vi "record.vi"(0 "Camera in":refnum<class "Camera.lvclass">, 5 "num_images":u32=1, 7 "record_mode":T1(ring), 9 "file_path":path, 11 "error in (no error)":errorcluster, 12 "wFlags":u16 format="%04x") -> (4 "Camera out":refnum<class "Camera.lvclass">, 15 "error out":errorcluster)   [LabVIEW 2019, in "Camera.lvclass"]
doc: "Creates, configures, and starts a new recorder instance. The entire camera configuration must be\nset before calling record.vi. The VI's for getting and setting delay/exposure time are the only exception.\nThese functions have no effect on the recorder object and can be called during the recording."
uses:
  Camera.lvclass
  Camera.lvclass/Camera.ctl
  pco.recorder/Recorder.lvlib
  pco.sdk/RecordingControl/RecordingControl.lvlib
  pco.sdk/ImageSensor/ImageSensor.lvlib
  pco.convert/Convert.lvlib
panel:
  out "filemode_no_overwrite":bool
  out "blocking_int":bool
  out "recType_int":u16
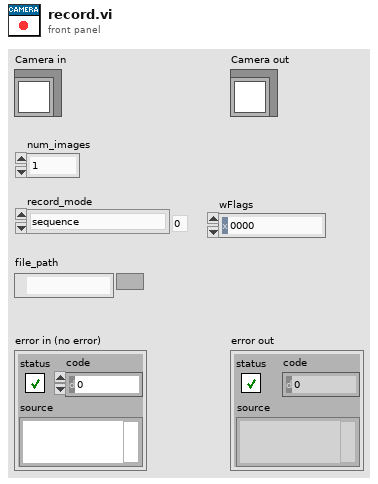
[diagram p1: front panel]
types:
  T1 = enum16{"sequence", "sequence non blocking", "ring buffer", "fifo", "tif", "multitif", "pcoraw", "b16", "dicom", "multidicom", "camram_ring", "camram_segment"}
  T2 = map{enum16{"Undefined", "Mono8", "Mono16", "BGRA8", "RGBA8", "BGRA16", "RGBA16", "CompressedMono8"}, bool}
  T3 = cluster{"wSensorTypeDESC":u16, "wSensorSubTypeDESC":u16, "wMaxHorzResStdDESC":u16, "wMaxVertResStdDESC":u16, "wMaxHorzResExtDESC":u16, "wMaxVertResExtDESC":u16, "wDynResDESC":u16, "wMaxBinHorzDESC":u16, "wBinHorzSteppingDESC":u16, "wMaxBinVertDESC":u16, "wBinVertSteppingDESC":u16, "wRoiHorStepsDESC":u16, "wRoiVertStepsDESC":u16, "wNumADCsDESC":u16, "wMinSizeHorzDESC":u16, "dwPixelRateDESC":u32[], "wConvFactDESC":u16[], "sCoolingSetpoints":i16[], "wSoftRoiHorStepsDESC":u16, "wSoftRoiVertStepsDESC":u16, "wIRDESC":u16, "wMinSizeVertDESC":u16, "dwMinDelayDESC":u32, "dwMaxDelayDESC":u32, "dwMinDelayStepDESC":u32, "dwMinExposureDESC":u32, "dwMaxExposureDESC":u32, "dwMinExposureStepDESC":u32, "dwMinDelayIRDESC":u32, "dwMaxDelayIRDESC":u32, "dwMinExposureIRDESC":u32, "dwMaxExposureIRDESC":u32, "wTimeTableDESC":u16, "wDoubleImageDESC":u16, "sMinCoolSetDESC":i16, "sMaxCoolSetDESC":i16, "sDefaultCoolSetDESC":i16, "wPowerDownModeDESC":u16, "wOffsetRegulationDESC":u16, "wColorPatternDESC":u16, "wPatternTypeDESC":u16, "wNumCoolingSetpoints":u16, "dwGeneralCapsDESC1":u32, "dwGeneralCapsDESC2":u32, "dwExtSyncFrequency":u32[], "dwGeneralCapsDESC3":u32, "dwGeneralCapsDESC4":u32}
  T4 = cluster{"iConversionFactor":i32, "iDataBits":i32, "iSensorInfoBits":i32, "iDarkOffset":i32, "strColorCoeff":dbl[], "iCamNum":i32, "hCamera":u64}
  T5 = map{enum16{"Undefined", "Mono8", "Mono16", "BGRA8", "RGBA8", "BGRA16", "RGBA16", "CompressedMono8"}, u64}
  T6 = enum16{"Undefined", "Mono8", "Mono16", "BGRA8", "RGBA8", "BGRA16", "RGBA16", "CompressedMono8"}
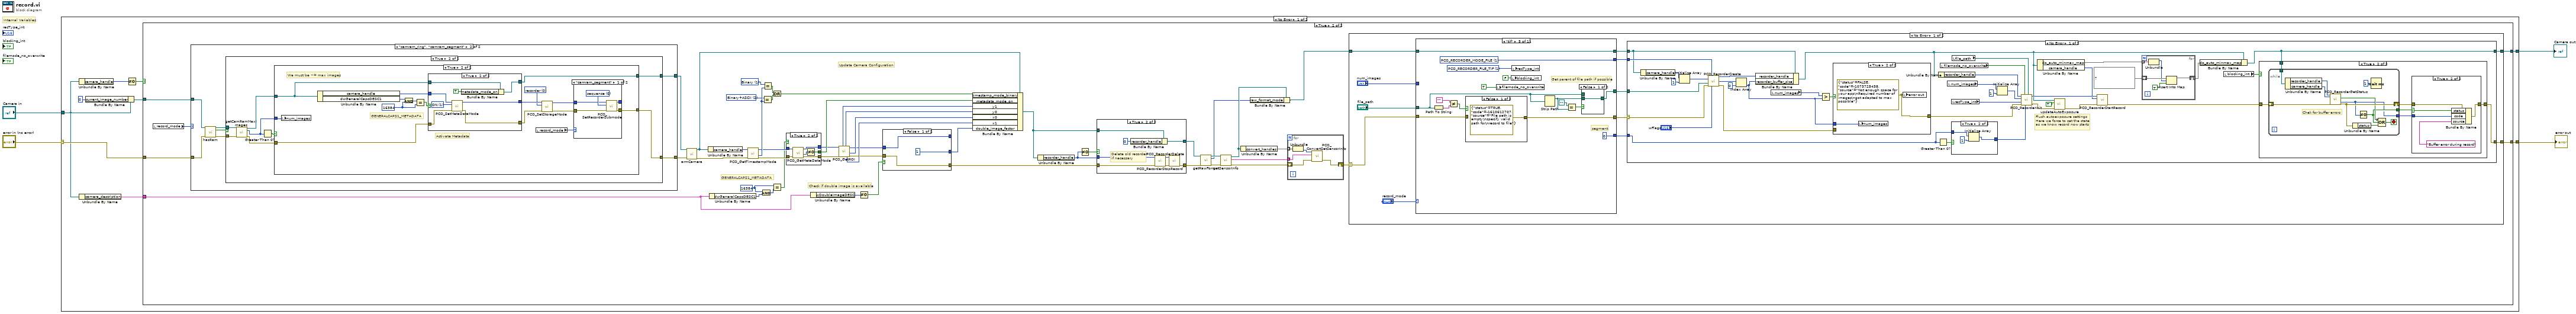
[diagram p0: block diagram]
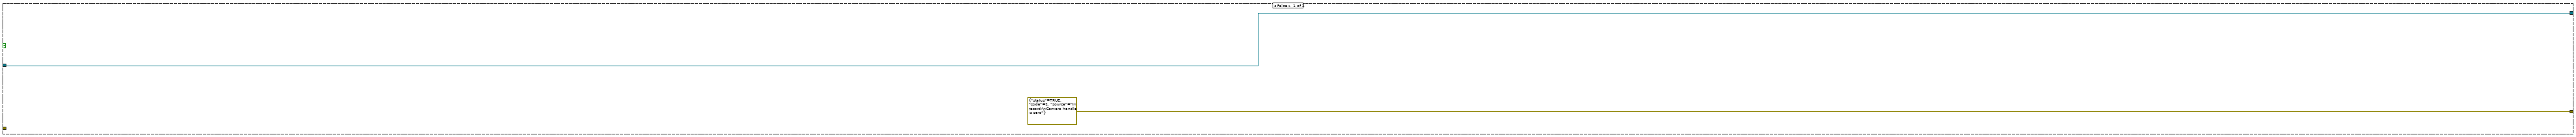
[diagram p2: hidden frame]
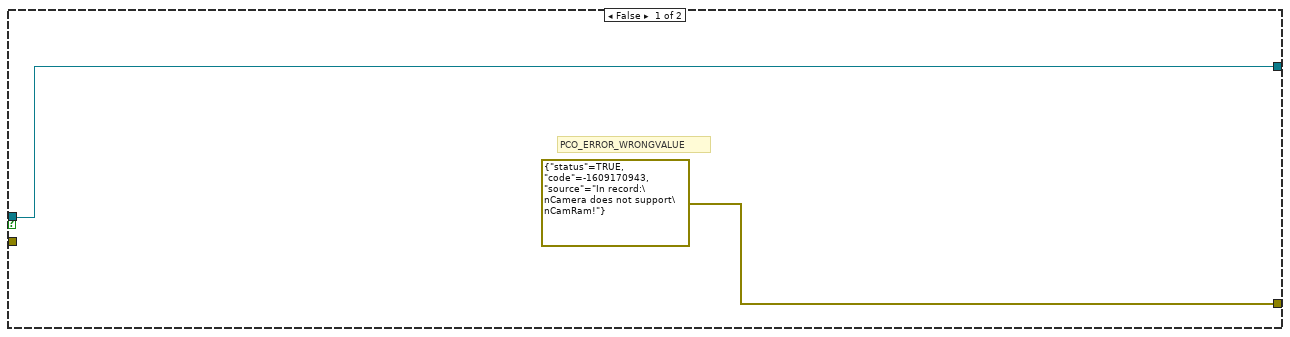
[diagram p4: hidden frame]
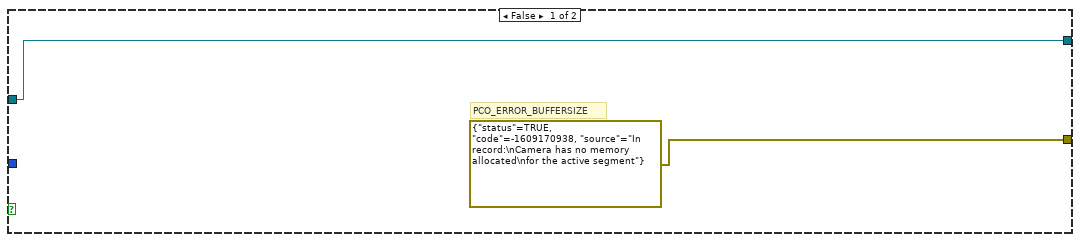
[diagram p5: hidden frame]
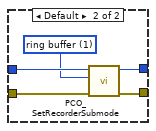
[diagram p6: hidden frame]
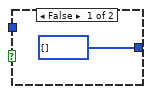
[diagram p8: hidden frame]
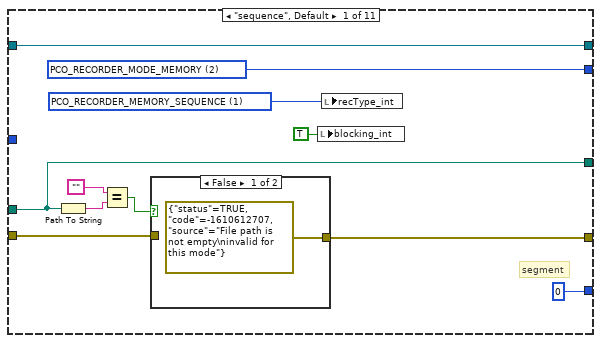
[diagram p13: hidden frame]
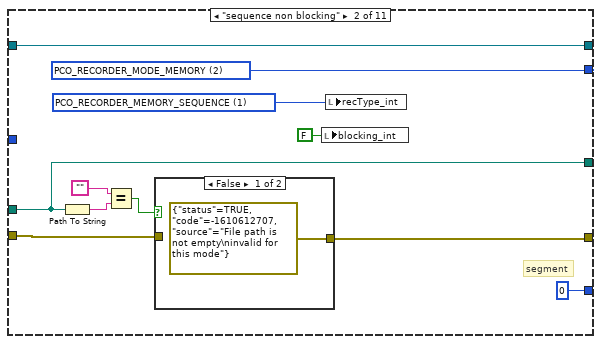
[diagram p15: hidden frame]
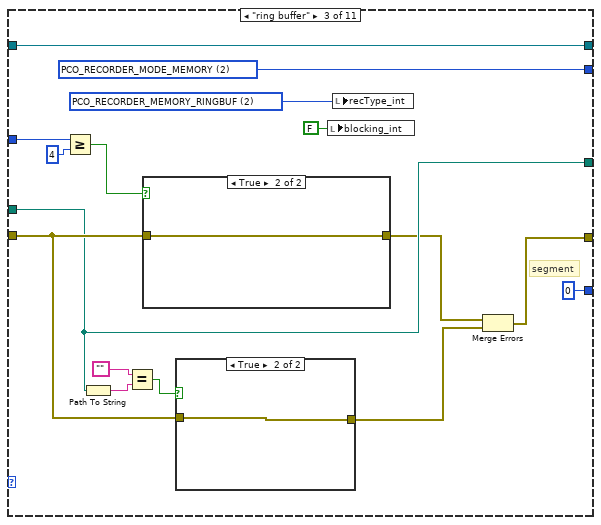
[diagram p17: hidden frame]
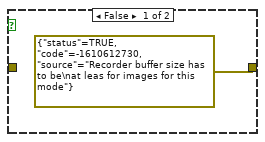
[diagram p18: hidden frame]
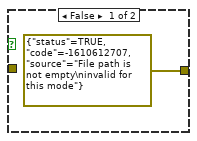
[diagram p19: hidden frame]
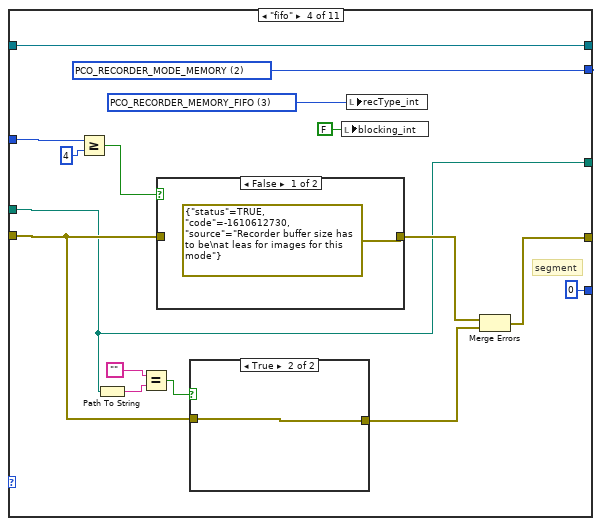
[diagram p20: hidden frame]
diagram:
  # "Internal Variables"
  n1 = case shown="No Error" "error in (no error)" {
    selector: "error in (no error)" -> [w9 w453]
    tunnel: [w12 w453] -> w3
    tunnel: [w11 w452] -> w1
    tunnel: "Camera in" -> [w7 w452]
    frame No Error {
      n2 = Unbundle By Name(w7) -> ("camera_handle"=w10:u64)
      n3 = Unbundle By Name(w7) -> ("camera_description"=w8:T3)
      n4 = Bundle By Name(cluster=w7, "current_image_number"=u32 0) -> (w6:refnum<class "Camera.lvclass">)
      n5 = Not Equal To 0?(x=w10) -> (x != 0?=w13:bool)
      n6 = case shown="True" w13 {
        tunnel: [errorcluster {"status"=TRUE, "code"=1, "source"="In record:\nCamera handle is zero"} ("error constant") w32] -> w12
        tunnel: w9 -> [_ w29]
        tunnel: w6 -> [w14 w27]
        tunnel: [w14 w31] -> w11
        tunnel: w8 -> [_ w45]
        frame False {
        }
        frame True {
          w54 = u32 16384 ("dwGeneralCapsDESC1")
          w62 = u16 2 items=["OFF", "Binary", "Binary+ASCII", "ASCII"] ("wTimeStampMode")
          w64 = u16 1 items=["OFF", "Binary", "Binary+ASCII", "ASCII"] ("wTimeStampMode")
          # "Update Camera Configuration"
          # "Check if double image is available"
          # "GENERALCAPS1_METADATA"
          n7 = local read "record_mode"() -> (w30:T1)
          n8 = case shown="\"camram_ring\", \"camram_segment\"" w30 {
            tunnel: w29 -> [w67 w72]
            tunnel: [w67 w68] -> w28
            tunnel: w27 -> [w66 w73]
            tunnel: [w66 w69] -> w18
            frame Default {
            }
            frame "camram_ring", "camram_segment" {
              n9 = call-dynamic "hasRam.vi"("Camera in"=w73, "error in (no error)"=w72) -> ("Camera out"=w70:refnum<class "Camera.lvclass">, "hasRam"=w74:bool, "error out"=w71:errorcluster)  [unwired: 11 in]
              n10 = case shown="True" w74 {
                tunnel: w71 -> [_ w83]
                tunnel: w70 -> [w76 w84]
                tunnel: [w76 w78] -> w69
                tunnel: [errorcluster {"status"=TRUE, "code"=-1609170943, "source"="In record:\nCamera does not support\nCamRam!"} ("error constant") w77] -> w68
                frame False {
                  # "PCO_ERROR_WRONGVALUE"
                }
                frame True {
                  n11 = call-dynamic "getCamRamMaxImages.vi"("Camera in"=w84, "error in (no error)"=w83) -> ("Camera out"=w80:refnum<class "Camera.lvclass">, "max_images"=w79:u32, "error out"=w81:errorcluster)  [unwired: 11 in]
                  n12 = Greater Than 0?(x=w79) -> (x > 0?=w82:bool)
                  n13 = case shown="True" w82 {
                    tunnel: w81 -> [_ w97]
                    tunnel: w80 -> [w86 w96]
                    tunnel: w79 -> [_ w87]
                    tunnel: [w86 w89] -> w78
                    tunnel: [errorcluster {"status"=TRUE, "code"=-1609170938, "source"="In record:\nCamera has no memory allocated\nfor the active segment"} ("error constant") w88] -> w77
                    frame False {
                      # "PCO_ERROR_BUFFERSIZE"
                    }
                    frame True {
                      w93 = u16 0 items=["recorder", "FIFO buffer"] ("wStorageMode")
                      w101 = u32 16384 ("y")
                      # "Activate Metadata"
                      # "GENERALCAPS1_METADATA"
                      # "We must be <= max images"
                      n14 = local write "num_images"(w87) -> ()
                      n15 = Unbundle By Name(w96) -> ("camera_handle"=w98:u64, "dwGeneralCapsDESC1"=w100:u32)
                      n16 = And(x=w100, y=w101) -> (x .and. y?=w102:u32)
                      n17 = Equal?(x=w102, y=w101) -> (x = y?=w99:bool)
                      n18 = case shown="True" w99 {
                        tunnel: w98 -> [w114 w123]
                        tunnel: w97 -> [w115 w122]
                        tunnel: w96 -> [w113 w120]
                        tunnel: [w113 w118] -> w89
                        tunnel: [w115 w117] -> w94
                        tunnel: [w114 w116] -> w95
                        frame False {
                        }
                        frame True {
                          w121 = u16 1 items=["OFF", "ON"] ("wMetaDataMode")
                          n19 = call "PCO_SetMetaDataMode.vi"("error in (no error)"=w122, "wMetaDataMode"=w121, "ph"=w123) -> ("error out"=w117:errorcluster, "ph out"=w116:u64)  [unwired: 4 in, 3 out]
                          n20 = Bundle By Name(cluster=w120, "metadata_mode_on"=TRUE) -> (w118:refnum<class "Camera.lvclass">)
                        }
                      }
                      n21 = local read "record_mode"() -> (w92:T1)
                      n22 = call "PCO_SetStorageMode.vi"("error in (no error)"=w94, "wStorageMode"=w93, "ph"=w95) -> ("error out"=w91:errorcluster, "ph out"=w90:u64)  [unwired: 6 in, 1 out]
                      n23 = case shown="\"camram_segment\"" w92 {
                        tunnel: w91 -> [w105 w111]
                        tunnel: w90 -> [w106 w112]
                        tunnel: [w104 w109] -> _
                        tunnel: [w103 w108] -> w88
                        frame "camram_segment" {
                          w107 = u16 0 items=["sequence", "ring buffer"] ("wRecSubmode")
                          n24 = call "PCO_SetRecorderSubmode.vi"("error in (no error)"=w105, "wRecSubmode"=w107, "ph"=w106) -> ("error out"=w103:errorcluster, "ph out"=w104:u64)  [unwired: 6 in, 1 out]
                        }
                        frame Default {
                          w110 = u16 1 items=["sequence", "ring buffer"] ("wRecSubmode")
                          n25 = call "PCO_SetRecorderSubmode.vi"("error in (no error)"=w111, "wRecSubmode"=w110, "ph"=w112) -> ("error out"=w108:errorcluster, "ph out"=w109:u64)  [unwired: 6 in, 1 out]
                        }
                      }
                    }
                  }
                }
              }
            }
          }
          n26 = call-dynamic "armCamera.vi"("Camera in"=w18, "error in (no error)"=w28) -> ("Camera out"=w16:refnum<class "Camera.lvclass">, "error out"=w65:errorcluster)  [unwired: 12 in]
          n27 = Unbundle By Name(w16) -> ("camera_handle"=w17:u64)
          n28 = Unbundle By Name(w45) -> ("dwGeneralCapsDESC1"=w56:u32)
          n29 = call "PCO_GetTimestampMode.vi"("error in (no error)"=w65, "ph"=w17) -> ("error out"=w57:errorcluster, "wTimeStampMode"=w63:u16, "ph out"=w58:u64)  [unwired: 6 in, 1 out]
          n30 = And(x=w54, y=w56) -> (x .and. y?=w55:u32)
          n31 = Equal?(x=w62, y=w63) -> (x = y?=w61:bool)
          n32 = Equal?(x=w64, y=w63) -> (x = y?=w60:bool)
          n33 = Or(x=w60, y=w61) -> (x .or. y?=w59:bool)
          n34 = Equal?(x=w54, y=w55) -> (x = y?=w53:bool)
          n35 = case shown="True" w53 {
            tunnel: w58 -> [w443 w451]
            tunnel: w57 -> [w444 w450]
            tunnel: [w443 w449] -> w51
            tunnel: [w444 w448] -> w50
            tunnel: [FALSE w446] -> w52
            frame False {
            }
            frame True {
              n36 = call "PCO_GetMetaDataMode.vi"("error in (no error)"=w450, "ph"=w451) -> ("error out"=w448:errorcluster, "wMetaDataMode"=w447:u16, "ph out"=w449:u64)  [unwired: 4 in, 3 out]
              n37 = Not Equal To 0?(x=w447) -> (x != 0?=w446:bool)
            }
          }
          n38 = Unbundle By Name(w45) -> ("wDoubleImageDESC"=w44:u16)
          n39 = call "PCO_GetROI.vi"("error in (no error)"=w50, "ph"=w51) -> ("error out"=w42:errorcluster, "wRoiX0"=w47:u16, "ph out"=w41:u64, "wRoiX1"=w46:u16, "wRoiY0"=w49:u16, "wRoiY1"=w48:u16)  [unwired: 3 in, 1 out]
          n40 = Not Equal To 0?(x=w44) -> (x != 0?=w43:bool)
          n41 = case shown="False" w43 {
            tunnel: w42 -> [w431 w440]
            tunnel: w41 -> [w432 w439]
            tunnel: [u16 1 ("double_image_factor") w436] -> w40
            tunnel: [w431 w435] -> w39
            tunnel: [w432 w434] -> _
            frame False {
            }
            frame True {
              n42 = call "PCO_GetDoubleImageMode.vi"("error in (no error)"=w440, "ph"=w439) -> ("error out"=w435:errorcluster, "wDoubleImage"=w438:u16, "ph out"=w434:u64)  [unwired: 6 in, 1 out]
              n43 = Not Equal To 0?(x=w438) -> (x != 0?=w437:bool)
              n44 = case shown="True" w437 {
                tunnel: [u16 1 ("double_image_factor") u16 2 ("double_image_factor")] -> w436
                frame False {
                }
                frame True {
                }
              }
            }
          }
          n45 = Bundle By Name(cluster=w16, "timestamp_mode_binary"=w59, "metadata_mode_on"=w52, "y1"=w48, "y0"=w49, "x0"=w47, "x1"=w46, "double_image_factor"=w40) -> (w26:refnum<class "Camera.lvclass">)
          n46 = Unbundle By Name(w26) -> ("recorder_handle"=w37:u64)
          n47 = Not Equal To 0?(x=w37) -> (x != 0?=w38:bool)
          n48 = case shown="True" w38 {
            tunnel: w37 -> [_ w429]
            tunnel: w39 -> [w422 w430]
            tunnel: [w422 w426] -> w22
            tunnel: w26 -> [w421 w425]
            tunnel: [w421 w423] -> w23
            frame False {
            }
            frame True {
              # "Delete old recorder\nif necessary"
              n49 = Bundle By Name(cluster=w425, "recorder_handle"=u64 0) -> (w423:refnum<class "Camera.lvclass">)
              n50 = call "PCO_RecorderStopRecord.vi"("error in (no error)"=w430, "phRec"=w429) -> ("error out"=w428:errorcluster, "phRec out"=w427:u64)  [unwired: 7 in, 1 out]
              n51 = call "PCO_RecorderDelete.vi"("error in (no error)"=w428, "phRec"=w427) -> ("error out"=w426:errorcluster)  [unwired: 8 in, 1 out]
            }
          }
          n52 = call-dynamic "getRawFormat.vi"("Camera in"=w23, "error in (no error)"=w22) -> ("Camera out"=w25:refnum<class "Camera.lvclass">, "rawFormat"=w20:enum16{"Word", "Byte"}, "error out"=w24:errorcluster)  [unwired: 11 in]
          n53 = call-dynamic "getSensorInfo.vi"("error in (no error)"=w24, "Camera in"=w25) -> ("error out"=w34:errorcluster, "PCO_SensorInfo"=w35:T4, "Camera out"=w21:refnum<class "Camera.lvclass">)  [unwired: 7 in]
          n54 = Unbundle By Name(w21) -> ("convert_handles"=w36:T5)
          n55 = Bundle By Name(cluster=w21, "raw_format_mode"=w20) -> (w19:refnum<class "Camera.lvclass">)
          n56 = for {
            tunnel: w36 -> [w420] mode=indexing
            tunnel: w35 -> [w418]
            shift-right: [w416] -> w33
            shift-left: w34 -> [w417]
            n57 = Unbundle(w420) -> (w419:u64)  [unwired: 1 out]
            n58 = call "PCO_ConvertSetSensorInfo.vi"("error in (no error)"=w417, "strSensorInfo"=w418, "ph"=w419) -> ("error out"=w416:errorcluster)  [unwired: 6 in, 2 out]
          }
          n59 = case shown="No Error" w33 {
            selector: w33 -> [w128 w415]
            tunnel: [w125 w415] -> w32
            tunnel: w19 -> [w134 w414]
            tunnel: [w126 w414] -> w31
            frame No Error {
              n60 = case shown="\"tif\"" "record_mode" {
                tunnel: w134 -> [w218 w236 w247 w260 w284 w302 w321 w341 w361 w383 w404]
                tunnel: "file_path" -> [w217 w228 w243 w263 w283 w306 w325 w346 w366 w386 w406]
                tunnel: "num_images" -> [_ _ w254 w265 _ _ _ _ _ _ _]
                tunnel: [w214 w229 w240 w262 w282 w303 w324 w343 w363 w381 w399] -> w129
                tunnel: [w219 w227 w246 w261 w286 w301 w322 w342 w362 w384 w405] -> w131
                tunnel: [w218 w236 w247 w260 w284 w302 w321 w341 w361 w383 w401] -> w130
                tunnel: [w217 w228 w243 w263 w281 w304 w323 w344 w364 w382 w406] -> w127
                tunnel: w128 -> [w215 w230 w244 w264 w287 w305 w326 w345 w365 w385 w403]
                tunnel: [u16 0 u16 0 u16 0 u16 0 u16 0 u16 0 u16 0 u16 0 u16 0 u16 0 w400] -> w124
                frame "sequence", Default {
                  w219 = u16 2 items=["PCO_RECORDER_MODE_FILE"=1, "PCO_RECORDER_MODE_MEMORY"=2, "PCO_RECORDER_MODE_CAMRAM"=3] ("wRecMode")
                  w220 = u16 1 items=["PCO_RECORDER_MEMORY_SEQUENCE"=1, "PCO_RECORDER_MEMORY_RINGBUF"=2, "PCO_RECORDER_MEMORY_FIFO"=3] ("wRecType")
                  # "segment"
                  n61 = Path To String(path=w217) -> (string=w222:string)
                  n62 = Equal?(x="", y=w222) -> (x = y?=w216:bool)
                  n63 = case shown="False" w216 {
                    tunnel: w215 -> [_ w225]
                    tunnel: [errorcluster {"status"=TRUE, "code"=-1610612707, "source"="File path is not empty\ninvalid for this mode"} ("error constant") w225] -> w214
                    frame False {
                    }
                    frame True {
                    }
                  }
                  n64 = local write "blocking_int"(TRUE ("blocking_int")) -> ()
                  n65 = local write "recType_int"(w220) -> ()
                }
                frame "sequence non blocking" {
                  w227 = u16 2 items=["PCO_RECORDER_MODE_FILE"=1, "PCO_RECORDER_MODE_MEMORY"=2, "PCO_RECORDER_MODE_CAMRAM"=3] ("wRecMode")
                  w232 = u16 1 items=["PCO_RECORDER_MEMORY_SEQUENCE"=1, "PCO_RECORDER_MEMORY_RINGBUF"=2, "PCO_RECORDER_MEMORY_FIFO"=3] ("wRecType")
                  # "segment"
                  n66 = Path To String(path=w228) -> (string=w234:string)
                  n67 = Equal?(x="", y=w234) -> (x = y?=w231:bool)
                  n68 = case shown="False" w231 {
                    tunnel: w230 -> [_ w238]
                    tunnel: [errorcluster {"status"=TRUE, "code"=-1610612707, "source"="File path is not empty\ninvalid for this mode"} ("error constant") w238] -> w229
                    frame False {
                    }
                    frame True {
                    }
                  }
                  n69 = local write "blocking_int"(FALSE ("blocking_int")) -> ()
                  n70 = local write "recType_int"(w232) -> ()
                }
                frame "ring buffer" {
                  w246 = u16 2 items=["PCO_RECORDER_MODE_FILE"=1, "PCO_RECORDER_MODE_MEMORY"=2, "PCO_RECORDER_MODE_CAMRAM"=3] ("wRecMode")
                  w249 = u16 2 items=["PCO_RECORDER_MEMORY_SEQUENCE"=1, "PCO_RECORDER_MEMORY_RINGBUF"=2, "PCO_RECORDER_MEMORY_FIFO"=3] ("wRecType")
                  # "segment"
                  n71 = Greater Or Equal?(x=w254, y=u32 4) -> (x >= y?=w245:bool)
                  n72 = Path To String(path=w243) -> (string=w251:string)
                  n73 = Equal?(x="", y=w251) -> (x = y?=w248:bool)
                  n74 = case shown="True" w245 {
                    tunnel: w244 -> [_ w256]
                    tunnel: [errorcluster {"status"=TRUE, "code"=-1610612730, "source"="Recorder buffer size has to be\nat leas for images for this mode"} ("error constant") w256] -> w242
                    frame False {
                    }
                    frame True {
                    }
                  }
                  n75 = case shown="True" w248 {
                    tunnel: w244 -> [_ w258]
                    tunnel: [errorcluster {"status"=TRUE, "code"=-1610612707, "source"="File path is not empty\ninvalid for this mode"} ("error constant") w258] -> w241
                    frame False {
                    }
                    frame True {
                    }
                  }
                  n76 = local write "blocking_int"(FALSE ("blocking_int")) -> ()
                  n77 = local write "recType_int"(w249) -> ()
                  n78 = Merge Errors(w242, w241) -> (w240:errorcluster)
                }
                frame "fifo" {
                  w261 = u16 2 items=["PCO_RECORDER_MODE_FILE"=1, "PCO_RECORDER_MODE_MEMORY"=2, "PCO_RECORDER_MODE_CAMRAM"=3] ("wRecMode")
                  w270 = u16 3 items=["PCO_RECORDER_MEMORY_SEQUENCE"=1, "PCO_RECORDER_MEMORY_RINGBUF"=2, "PCO_RECORDER_MEMORY_FIFO"=3] ("wRecType")
                  # "segment"
                  n79 = Greater Or Equal?(x=w265, y=u32 4) -> (x >= y?=w268:bool)
                  n80 = Path To String(path=w263) -> (string=w272:string)
                  n81 = Equal?(x="", y=w272) -> (x = y?=w269:bool)
                  n82 = case shown="False" w268 {
                    tunnel: w264 -> [_ w276]
                    tunnel: [errorcluster {"status"=TRUE, "code"=-1610612730, "source"="Recorder buffer size has to be\nat leas for images for this mode"} ("error constant") w276] -> w267
                    frame False {
                    }
                    frame True {
                    }
                  }
                  n83 = case shown="True" w269 {
                    tunnel: w264 -> [_ w278]
                    tunnel: [errorcluster {"status"=TRUE, "code"=-1610612707, "source"="File path is not empty\ninvalid for this mode"} ("error constant") w278] -> w266
                    frame False {
                    }
                    frame True {
                    }
                  }
                  n84 = local write "blocking_int"(FALSE ("blocking_int")) -> ()
                  n85 = local write "recType_int"(w270) -> ()
                  n86 = Merge Errors(w267, w266) -> (w262:errorcluster)
                }
                frame "tif" {
                  w285 = u16 1 items=["PCO_RECORDER_FILE_TIF"=1, "PCO_RECORDER_FILE_MULTITIF"=2, "PCO_RECORDER_FILE_PCORAW"=3, "PCO_RECORDER_FILE_B16"=4, "PCO_RECORDER_FILE_DICOM"=5, "PCO_RECORDER_FILE_MULTIDICOM"=6] ("wRecType")
                  w286 = u16 1 items=["PCO_RECORDER_MODE_FILE"=1, "PCO_RECORDER_MODE_MEMORY"=2, "PCO_RECORDER_MODE_CAMRAM"=3] ("wRecMode")
                  # "segment"
                  # "Get parent of file path if possible"
                  n87 = Path To String(path=w283) -> (string=w290:string)
                  n88 = Not Equal?(x="", y=w290) -> (x != y?=w288:bool)
                  n89 = case shown="False" w288 {
                    tunnel: w287 -> [_ w296]
                    tunnel: [errorcluster {"status"=TRUE, "code"=-1610612707, "source"="File path is empty\nspecify valid path for\nrecord to file"} ("error constant") w296] -> w282
                    frame False {
                    }
                    frame True {
                    }
                  }
                  n90 = local write "filemode_no_overwrite"(TRUE ("blocking_int")) -> ()
                  n91 = local write "blocking_int"(FALSE ("blocking_int")) -> ()
                  n92 = local write "recType_int"(w285) -> ()
                  n93 = Strip Path(path=w283) -> (stripped path=w292:path)  [unwired: 1 out]
                  n94 = Equal?(x=path "", y=w292) -> (x = y?=w293:bool)
                  n95 = case shown="False" w293 {
                    tunnel: w292 -> [w297 _]
                    tunnel: w283 -> [_ w298]
                    tunnel: [w297 w298] -> w281
                    frame False {
                    }
                    frame True {
                    }
                  }
                }
                frame "multitif" {
                  w307 = u16 2 items=["PCO_RECORDER_FILE_TIF"=1, "PCO_RECORDER_FILE_MULTITIF"=2, "PCO_RECORDER_FILE_PCORAW"=3, "PCO_RECORDER_FILE_B16"=4, "PCO_RECORDER_FILE_DICOM"=5, "PCO_RECORDER_FILE_MULTIDICOM"=6] ("wRecType")
                  w301 = u16 1 items=["PCO_RECORDER_MODE_FILE"=1, "PCO_RECORDER_MODE_MEMORY"=2, "PCO_RECORDER_MODE_CAMRAM"=3] ("wRecMode")
                  # "segment"
                  # "Get parent of file path if possible"
                  n96 = Path To String(path=w306) -> (string=w310:string)
                  n97 = Not Equal?(x="", y=w310) -> (x != y?=w308:bool)
                  n98 = case shown="False" w308 {
                    tunnel: w305 -> [_ w316]
                    tunnel: [errorcluster {"status"=TRUE, "code"=-1610612707, "source"="File path is empty\nspecify valid path for\nrecord to file"} ("error constant") w316] -> w303
                    frame False {
                    }
                    frame True {
                    }
                  }
                  n99 = local write "filemode_no_overwrite"(TRUE ("blocking_int")) -> ()
                  n100 = local write "blocking_int"(FALSE ("blocking_int")) -> ()
                  n101 = local write "recType_int"(w307) -> ()
                  n102 = Strip Path(path=w306) -> (stripped path=w312:path)  [unwired: 1 out]
                  n103 = Equal?(x=path "", y=w312) -> (x = y?=w313:bool)
                  n104 = case shown="False" w313 {
                    tunnel: w312 -> [w317 _]
                    tunnel: w306 -> [_ w318]
                    tunnel: [w317 w318] -> w304
                    frame False {
                    }
                    frame True {
                    }
                  }
                }
                frame "pcoraw" {
                  w327 = u16 3 items=["PCO_RECORDER_FILE_TIF"=1, "PCO_RECORDER_FILE_MULTITIF"=2, "PCO_RECORDER_FILE_PCORAW"=3, "PCO_RECORDER_FILE_B16"=4, "PCO_RECORDER_FILE_DICOM"=5, "PCO_RECORDER_FILE_MULTIDICOM"=6] ("wRecType")
                  w322 = u16 1 items=["PCO_RECORDER_MODE_FILE"=1, "PCO_RECORDER_MODE_MEMORY"=2, "PCO_RECORDER_MODE_CAMRAM"=3] ("wRecMode")
                  # "segment"
                  # "Get parent of file path if possible"
                  n105 = Path To String(path=w325) -> (string=w330:string)
                  n106 = Not Equal?(x="", y=w330) -> (x != y?=w328:bool)
                  n107 = case shown="False" w328 {
                    tunnel: w326 -> [_ w336]
                    tunnel: [errorcluster {"status"=TRUE, "code"=-1610612707, "source"="File path is empty\nspecify valid path for\nrecord to file"} ("error constant") w336] -> w324
                    frame False {
                    }
                    frame True {
                    }
                  }
                  n108 = local write "filemode_no_overwrite"(TRUE ("blocking_int")) -> ()
                  n109 = local write "blocking_int"(FALSE ("blocking_int")) -> ()
                  n110 = local write "recType_int"(w327) -> ()
                  n111 = Strip Path(path=w325) -> (stripped path=w332:path)  [unwired: 1 out]
                  n112 = Equal?(x=path "", y=w332) -> (x = y?=w333:bool)
                  n113 = case shown="True" w333 {
                    tunnel: w332 -> [w337 _]
                    tunnel: w325 -> [_ w338]
                    tunnel: [w337 w338] -> w323
                    frame False {
                    }
                    frame True {
                    }
                  }
                }
                frame "b16" {
                  w347 = u16 4 items=["PCO_RECORDER_FILE_TIF"=1, "PCO_RECORDER_FILE_MULTITIF"=2, "PCO_RECORDER_FILE_PCORAW"=3, "PCO_RECORDER_FILE_B16"=4, "PCO_RECORDER_FILE_DICOM"=5, "PCO_RECORDER_FILE_MULTIDICOM"=6] ("wRecType")
                  w342 = u16 1 items=["PCO_RECORDER_MODE_FILE"=1, "PCO_RECORDER_MODE_MEMORY"=2, "PCO_RECORDER_MODE_CAMRAM"=3] ("wRecMode")
                  # "segment"
                  # "Get parent of file path if possible"
                  n114 = Path To String(path=w346) -> (string=w350:string)
                  n115 = Not Equal?(x="", y=w350) -> (x != y?=w348:bool)
                  n116 = case shown="False" w348 {
                    tunnel: w345 -> [_ w356]
                    tunnel: [errorcluster {"status"=TRUE, "code"=-1610612707, "source"="File path is empty\nspecify valid path for\nrecord to file"} ("error constant") w356] -> w343
                    frame False {
                    }
                    frame True {
                    }
                  }
                  n117 = local write "filemode_no_overwrite"(TRUE ("blocking_int")) -> ()
                  n118 = local write "blocking_int"(FALSE ("blocking_int")) -> ()
                  n119 = local write "recType_int"(w347) -> ()
                  n120 = Strip Path(path=w346) -> (stripped path=w352:path)  [unwired: 1 out]
                  n121 = Equal?(x=path "", y=w352) -> (x = y?=w353:bool)
                  n122 = case shown="True" w353 {
                    tunnel: w352 -> [w357 _]
                    tunnel: w346 -> [_ w358]
                    tunnel: [w357 w358] -> w344
                    frame False {
                    }
                    frame True {
                    }
                  }
                }
                frame "dicom" {
                  w367 = u16 5 items=["PCO_RECORDER_FILE_TIF"=1, "PCO_RECORDER_FILE_MULTITIF"=2, "PCO_RECORDER_FILE_PCORAW"=3, "PCO_RECORDER_FILE_B16"=4, "PCO_RECORDER_FILE_DICOM"=5, "PCO_RECORDER_FILE_MULTIDICOM"=6] ("wRecType")
                  w362 = u16 1 items=["PCO_RECORDER_MODE_FILE"=1, "PCO_RECORDER_MODE_MEMORY"=2, "PCO_RECORDER_MODE_CAMRAM"=3] ("wRecMode")
                  # "segment"
                  # "Get parent of file path if possible"
                  n123 = Path To String(path=w366) -> (string=w370:string)
                  n124 = Not Equal?(x="", y=w370) -> (x != y?=w368:bool)
                  n125 = case shown="False" w368 {
                    tunnel: w365 -> [_ w376]
                    tunnel: [errorcluster {"status"=TRUE, "code"=-1610612707, "source"="File path is empty\nspecify valid path for\nrecord to file"} ("error constant") w376] -> w363
                    frame False {
                    }
                    frame True {
                    }
                  }
                  n126 = local write "filemode_no_overwrite"(TRUE ("blocking_int")) -> ()
                  n127 = local write "blocking_int"(FALSE ("blocking_int")) -> ()
                  n128 = local write "recType_int"(w367) -> ()
                  n129 = Strip Path(path=w366) -> (stripped path=w372:path)  [unwired: 1 out]
                  n130 = Equal?(x=path "", y=w372) -> (x = y?=w373:bool)
                  n131 = case shown="True" w373 {
                    tunnel: w372 -> [w377 _]
                    tunnel: w366 -> [_ w378]
                    tunnel: [w377 w378] -> w364
                    frame False {
                    }
                    frame True {
                    }
                  }
                }
                frame "multidicom" {
                  w387 = u16 6 items=["PCO_RECORDER_FILE_TIF"=1, "PCO_RECORDER_FILE_MULTITIF"=2, "PCO_RECORDER_FILE_PCORAW"=3, "PCO_RECORDER_FILE_B16"=4, "PCO_RECORDER_FILE_DICOM"=5, "PCO_RECORDER_FILE_MULTIDICOM"=6] ("wRecType")
                  w384 = u16 1 items=["PCO_RECORDER_MODE_FILE"=1, "PCO_RECORDER_MODE_MEMORY"=2, "PCO_RECORDER_MODE_CAMRAM"=3] ("wRecMode")
                  # "segment"
                  # "Get parent of file path if possible"
                  n132 = Path To String(path=w386) -> (string=w390:string)
                  n133 = Not Equal?(x="", y=w390) -> (x != y?=w388:bool)
                  n134 = case shown="False" w388 {
                    tunnel: w385 -> [_ w396]
                    tunnel: [errorcluster {"status"=TRUE, "code"=-1610612707, "source"="File path is empty\nspecify valid path for\nrecord to file"} ("error constant") w396] -> w381
                    frame False {
                    }
                    frame True {
                    }
                  }
                  n135 = local write "filemode_no_overwrite"(TRUE ("blocking_int")) -> ()
                  n136 = local write "blocking_int"(FALSE ("blocking_int")) -> ()
                  n137 = local write "recType_int"(w387) -> ()
                  n138 = Strip Path(path=w386) -> (stripped path=w392:path)  [unwired: 1 out]
                  n139 = Equal?(x=path "", y=w392) -> (x = y?=w393:bool)
                  n140 = case shown="True" w393 {
                    tunnel: w392 -> [w397 _]
                    tunnel: w386 -> [_ w398]
                    tunnel: [w397 w398] -> w382
                    frame False {
                    }
                    frame True {
                    }
                  }
                }
                frame "camram_ring", "camram_segment" {
                  w405 = u16 3 items=["PCO_RECORDER_MODE_FILE"=1, "PCO_RECORDER_MODE_MEMORY"=2, "PCO_RECORDER_MODE_CAMRAM"=3] ("wRecMode")
                  w408 = u16 1 items=["PCO_RECORDER_CAMRAM_SEQUENTIAL"=1, "PCO_RECORDER_CAMRAM_SINGLE_IMAGE"=2] ("wRecType")
                  n141 = call-dynamic "getCamRamSegment.vi"("Camera in"=w404, "error in (no error)"=w403) -> ("Camera out"=w401:refnum<class "Camera.lvclass">, "segment"=w400:u16, "error out"=w402:errorcluster)  [unwired: 11 in]
                  n142 = Path To String(path=w406) -> (string=w411:string)
                  n143 = Equal?(x="", y=w411) -> (x = y?=w410:bool)
                  n144 = case shown="False" w410 {
                    tunnel: w402 -> [_ w413]
                    tunnel: [errorcluster {"status"=TRUE, "code"=-1610612707, "source"="File path is not empty\ninvalid for this mode"} ("error constant") w413] -> w399
                    frame False {
                    }
                    frame True {
                    }
                  }
                  n145 = local write "blocking_int"(FALSE ("blocking_int")) -> ()
                  n146 = local write "recType_int"(w408) -> ()
                }
              }
              n147 = case shown="No Error" w129 {
                selector: w129 -> [w167 w211]
                tunnel: [w149 w211] -> w125
                tunnel: w130 -> [w148 w212]
                tunnel: [w144 w212] -> w126
                tunnel: w131 -> [w168 _]
                tunnel: w127 -> [w166 _]
                tunnel: w124 -> [w141 _]
                frame No Error {
                  # "Flush autoexposure settings\nHere we force to set the state\nas we know record now starts"
                  n148 = Unbundle By Name(w148) -> ("camera_handle"=w173:u64)
                  n149 = Initialize Array(w173, 1 ("dimension size")) -> (w172:u64[])
                  n150 = call "PCO_RecorderCreate.vi"("wRecMode"=w168, "phCamArr"=w172, "szDrive"=w166, "error in (no error)"=w167, "wFlags"="wFlags") -> ("phRec out"=w169:u64, "dwMaxImgCountArr"=w170:u32[], "error out"=w160:errorcluster)  [unwired: 7 in, 1 out]
                  n151 = Index Array(array=w170, index=0) -> (element=w163:u32)
                  n152 = Bundle By Name(cluster=w148, "recorder_handle"=w169, "recorder_buffer_size"=w163) -> (w137:refnum<class "Camera.lvclass">)
                  n153 = local read "num_images"() -> (w165:u32)
                  n154 = Greater?(x=w165, y=w163) -> (0:w164:bool)
                  n155 = case shown="True" w164 {
                    tunnel: w163 -> [_ w210]
                    tunnel: w160 -> [w208 _]
                    tunnel: [w208 w209] -> w159
                    frame False {
                    }
                    frame True {
                      w209 = errorcluster {"status"=FALSE, "code"=-1073725438, "source"="Not enough space for your app\nRequired number of images\ngot adapted to max possible"} ("error constant")
                      n156 = local write "num_images"(w210) -> ()
                      n157 = local write "error out"(w209) -> ()
                    }
                  }
                  n158 = Greater Than 0?(x=w141) -> (x > 0?=w143:bool)
                  n159 = Unbundle By Name(w137) -> ("recorder_handle"=w162:u64)
                  n160 = local read "filemode_no_overwrite"() -> (w154:bool)
                  n161 = local read "num_images"() -> (w158:u32)
                  n162 = local read "recType_int"() -> (w156:u16)
                  n163 = case shown="True" w143 {
                    tunnel: [u16[] [] ("wRamSegmentArr") w176] -> w142
                    tunnel: w141 -> [_ w177]
                    frame False {
                    }
                    frame True {
                      n164 = Initialize Array(w177, 1 ("dimension size")) -> (w176:u16[])
                    }
                  }
                  n165 = local read "file_path"() -> (w155:path)
                  n166 = Initialize Array(w158, 1 ("dimension size")) -> (w157:u32[])
                  n167 = call "PCO_RecorderInit.vi"("szFilePath"=w155, "wRamSegmentArr"=w142, "noOverwrite"=w154, "error in (no error)"=w159, "wType"=w156, "dwImgCountArr"=w157, "phRec"=w162) -> ("error out"=w140:errorcluster, "phRec out"=w153:u64)  [unwired: 2 in, 1 out]
                  n168 = Unbundle By Name(w137) -> ("do_auto_minmax_map"=w147:T2, "camera_handle"=w152:u64)
                  n169 = call "updateAutoExposure.vi"("error in (no error)"=w140, "force"=TRUE, "Camera in"=w137) -> ("error out"=w139:errorcluster)  [unwired: 7 in, 1 out]
                  n170 = call "PCO_RecorderStartRecord.vi"("error in (no error)"=w139, "phCam"=w152, "phRec"=w153) -> ("error out"=w150:errorcluster)  [unwired: 6 in, 2 out]
                  n171 = for {
                    tunnel: w147 -> [w183] mode=indexing
                    shift-right: [w179] -> w145
                    shift-left: T2 {} ("do_auto_minmax_map") -> [w182]
                    n172 = Unbundle(w183) -> (w181:T6)  [unwired: 1 out]
                    n173 = Insert Into Map(map in=w182, key=w181, value=TRUE ("status")) -> (map out=w179:T2)  [unwired: 2 out]
                  }
                  n174 = Bundle By Name(cluster=w137, "do_auto_minmax_map"=w145) -> (w144:refnum<class "Camera.lvclass">)
                  n175 = local read "blocking_int"() -> (w151:bool)
                  n176 = case shown="True" w151 {
                    tunnel: w150 -> [w184 w190]
                    tunnel: w144 -> [_ w189]
                    tunnel: [w184 w186] -> w149
                    frame False {
                    }
                    frame True {
                      n177 = while {
                        shift-right: [w201] -> w187
                        shift-left: w190 -> [w204]
                        tunnel: w189 -> [w207]
                        tunnel: [w198] -> w188
                        tunnel: [w197] -> w185
                        stop <- w202 stop-if-true
                        # "Chek for buffer errors"
                        n178 = Unbundle By Name(w207) -> ("recorder_handle"=w206:u64, "camera_handle"=w205:u64)
                        n179 = call "PCO_RecorderGetStatus.vi"("phRec"=w206, "phCam"=w205, "error in (no error)"=w204) -> ("bIsRunning"=w199:bool, "dwLastError"=w197:u32, "error out"=w201:errorcluster)  [unwired: 5 in, 9 out]
                        n180 = Unbundle By Name(w201) -> ("status"=w203:bool)
                        n181 = Not Equal To 0?(x=w197) -> (x != 0?=w198:bool)
                        n182 = Wait (ms)(milliseconds to wait=u32 1) -> ()  [unwired: 1 out]
                        n183 = Compound Arithmetic op=OR(invert w199, w198, w203) -> (w202:bool)
                      }
                      n184 = case shown="True" w188 {
                        selector: w188 -> [_ w193]
                        tunnel: w187 -> [w191 w196]
                        tunnel: [w191 w194] -> w186
                        tunnel: w185 -> [_ w195]
                        frame False {
                        }
                        frame True {
                          n185 = Bundle By Name(cluster=w196, "status"=w193, "code"=w195, "source"="Buffer error during record") -> (w194:errorcluster)
                        }
                      }
                    }
                  }
                }
                frame Error {
                }
              }
            }
            frame Error {
            }
          }
        }
      }
    }
    frame Error {
    }
  }
  "error out" <- w3
  "Camera out" <- w1
